vi "Configure Trigger.vi"   [LabVIEW 2015, in "Tektronix 7000 Series.lvlib"]
doc: "Configures trigger settings for an oscilloscope."
uses:
  <instrlib>/Tektronix 7000 Series/Tektronix 7000 Series.lvlib
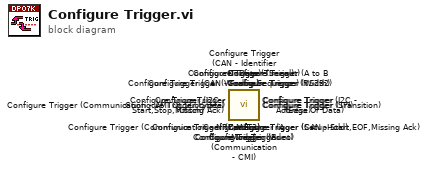
[diagram p0: block diagram]
diagram:
  n1 = call <instrlib>:"Configure Trigger (A Mode).vi"() -> ()  [unwired: 14 in, 2 out]
  n2 = call <instrlib>:"Configure Trigger (A to B Sequence).vi"() -> ()  [unwired: 14 in, 2 out]
  n3 = call <instrlib>:"Configure Trigger (I2C - Start,Stop,Missing Ack).vi"() -> ()  [unwired: 14 in, 2 out]
  n4 = call <instrlib>:"Configure Trigger (I2C - Address Or Data).vi"() -> ()  [unwired: 14 in, 2 out]
  n5 = call <instrlib>:"Configure Trigger (CAN - Frame).vi"() -> ()  [unwired: 14 in, 2 out]
  n6 = call <instrlib>:"Configure Trigger (CAN - Identifier Or Data).vi"() -> ()  [unwired: 14 in, 2 out]
  n7 = call <instrlib>:"Configure Trigger (CAN - Start,EOF,Missing Ack).vi"() -> ()  [unwired: 14 in, 2 out]
  n8 = call <instrlib>:"Configure Trigger (Communication - CMI).vi"() -> ()  [unwired: 14 in, 2 out]
  n9 = call <instrlib>:"Configure Trigger (Communication - NRZ,MLT3).vi"() -> ()  [unwired: 14 in, 2 out]
  n10 = call <instrlib>:"Configure Trigger (Communication - AMI Or Subtypes).vi"() -> ()  [unwired: 14 in, 2 out]
  n11 = call <instrlib>:"Configure Trigger (SPI).vi"() -> ()  [unwired: 14 in, 2 out]
  n12 = call <instrlib>:"Configure Trigger (RS232).vi"() -> ()  [unwired: 14 in, 2 out]
  n13 = call <instrlib>:"Configure Trigger (Serial).vi"() -> ()  [unwired: 14 in, 2 out]
  n14 = call <instrlib>:"Configure Trigger (Video).vi"() -> ()  [unwired: 14 in, 2 out]
  n15 = call <instrlib>:"Configure Trigger (Window).vi"() -> ()  [unwired: 13 in, 3 out]
  n16 = call <instrlib>:"Configure Trigger (Transition).vi"() -> ()  [unwired: 13 in, 3 out]
  n17 = call <instrlib>:"Configure Trigger (SetupHold).vi"() -> ()  [unwired: 13 in, 3 out]
  n18 = call <instrlib>:"Configure Trigger (State).vi"() -> ()  [unwired: 14 in, 2 out]
  n19 = call <instrlib>:"Configure Trigger (Pattern).vi"() -> ()  [unwired: 14 in, 2 out]
  n20 = call <instrlib>:"Configure Trigger (Timeout).vi"() -> ()  [unwired: 13 in, 3 out]
  n21 = call <instrlib>:"Configure Trigger (Runt).vi"() -> ()  [unwired: 13 in, 3 out]
  n22 = call <instrlib>:"Configure Trigger (Width).vi"() -> ()  [unwired: 13 in, 3 out]
  n23 = call <instrlib>:"Configure Trigger (Glitch).vi"() -> ()  [unwired: 13 in, 3 out]
  n24 = call <instrlib>:"Configure Trigger (Edge).vi"() -> ()  [unwired: 14 in, 2 out]
